vi "PDT Batch.vi"() -> ()   [LabVIEW 2018]
uses:
  <vilib>/Utility/file.llb/Read Delimited Spreadsheet (string).vi
panel:
  in  "Batch PDT FilePath":path
  in  "PDT *.csv FilePath":path
  out "String":string
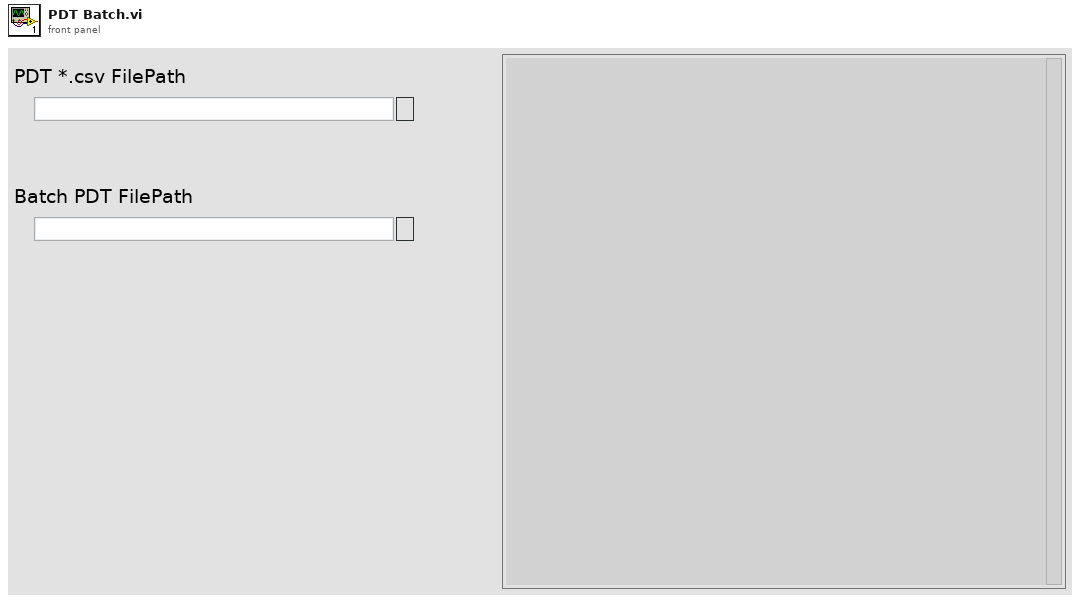
[diagram p1: front panel]
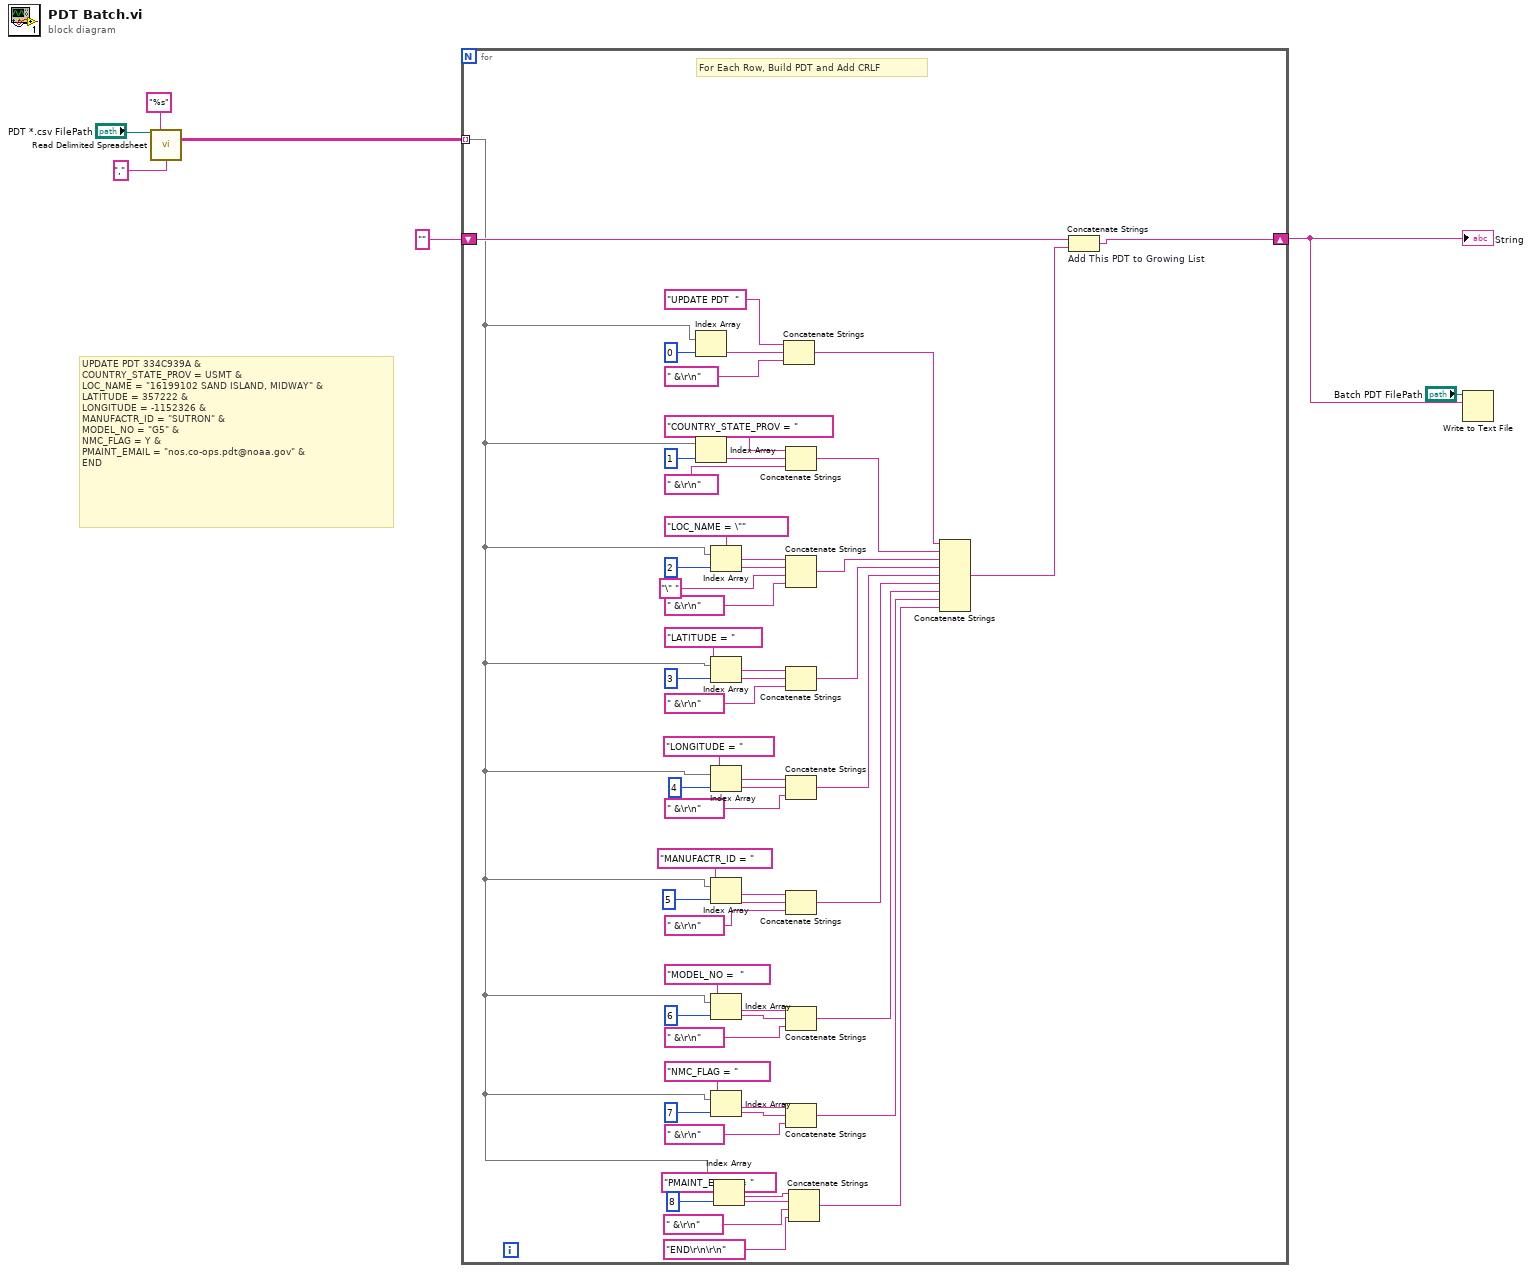
[diagram p0: block diagram]
diagram:
  # "UPDATE PDT 334C939A &\nCOUNTRY_STATE_PROV = USMT & \nLOC_NAME = \"16199102 SAND ISLAND, MIDWAY\" & \nLATITUDE = 357222 &\nLONGITUDE = -1152326 &\nMANUFACTR_ID = \"SUTRON\" & \nMODEL_NO = \"G5\" &\nNMC_FLAG = Y &\nPMAINT_EMAIL = \"nos.co-ops.pdt@noaa.gov\" & \nEND"
  n1 = call-poly <vilib>:"Read Delimited Spreadsheet.vi"("file path (dialog if empty)"="PDT *.csv FilePath", "format (%s)"="%s" ("format (%.3f)"), "delimiter (\\t)"="," ("delimiter (\\t)")) -> ("all rows"=w5:string[][])  [unwired: 7 in, 5 out]
  n2 = for {
    tunnel: w5 -> [w10] mode=indexing
    shift-right: [w43] -> w3
    shift-left: "" -> [w42]
    # "For Each Row, Build PDT and Add CRLF"
    n3 = Index Array(array=w10, index=0) -> (element=w56:string)
    n4 = Index Array(array=w10, index=1) -> (element=w35:string)
    n5 = Index Array(array=w10, index=2) -> (element=w54:string)
    n6 = Index Array(array=w10, index=3) -> (element=w31:string)
    n7 = Index Array(array=w10, index=4) -> (element=w28:string)
    n8 = Index Array(array=w10, index=5) -> (element=w39:string)
    n9 = Index Array(array=w10, index=6) -> (element=w51:string)
    n10 = Index Array(array=w10, index=7) -> (element=w12:string)
    n11 = Index Array(array=w10, index=8) -> (element=w48:string)
    n12 = Concatenate Strings("UPDATE PDT  ", w56, " &\r\n") -> (w37:string)
    n13 = Concatenate Strings("COUNTRY_STATE_PROV = ", w35, " &\r\n") -> (w33:string)
    n14 = Concatenate Strings("LOC_NAME = \"", w54, "\" ", " &\r\n") -> (w45:string)
    n15 = Concatenate Strings("LATITUDE = ", w31, " &\r\n") -> (w26:string)
    n16 = Concatenate Strings("LONGITUDE = ", w28, " &\r\n") -> (w25:string)
    n17 = Concatenate Strings("MANUFACTR_ID = ", w39, " &\r\n") -> (w24:string)
    n18 = Concatenate Strings("MODEL_NO =  ", w51, " &\r\n") -> (w16:string)
    n19 = Concatenate Strings("NMC_FLAG = ", w12, " &\r\n") -> (w8:string)
    n20 = Concatenate Strings("PMAINT_EMAIL = ", w48, " &\r\n", "END\r\n\r\n") -> (w9:string)
    n21 = Concatenate Strings(w37, w33, w45, w26, w25, w24, w16, w8, w9) -> (w44:string)
    n22 = Concatenate Strings "Add This PDT to Growing List"(w42, w44) -> (w43:string)
  }
  "String" <- w3
  n23 = Write to Text File(file (use dialog)="Batch PDT FilePath", text=w3) -> ()  [unwired: 2 in, 3 out]
